vi "START_ImagenPixel.vi"() -> ()   [LabVIEW 2021]
uses:
  <vilib>/vision/NI_Vision_Development_Module.lvlib
panel:
  out "secret_in_binary":string
  out "secret_length":i32
  in  "secret_to_introduce":string
  in  "number":u8
  out "Bolean_number":bool[](array[boolean])
  out "Blue Binary":string[][](array[string])
  out "Green Number":u8[][](array[numeric])
  out "Red Number":u8[][](array[numeric])
  out "Blue Number":u8[][](array[numeric])
  out "Green Binary":string[][](array[string])
  out "Red Binary":string[][](array[string])
  out "error":errorcluster
  out "Resolution":i32[](array[numeric])
  out "Image":T1(plugin-control)
  out "Color":u32(colorbox)
  # "Image Manipulation Example"
  # "Overview: This VI creates an images from a generater random value that represents pixel RGB intensity. Afterwards, it splits the generated image again and obtains the binary values of each individual pixel and plane. \n\nRemember, for our lab, you have to ONLY MODIFY THE PIXELS IN THE RED PLANE, otherwise, the decoder won't work.\n\n\nInstructions:\n1. Set some text in secret to introduce field and Run the VI.\n2. Red Number [0][0] --> represents the amount of red color in pixel [0][0]\n2. Green Number [0][0] --> represents the amount of green color in pixel [0][0]\n2. Blue Number [0][0] --> represents the amount of blue color in pixel [0][0]\n3. Red Number [0][1] --> represents the amount of red color in pixel [0][1]\n4.All arrays have 2 dimensions as the image is a matrix of pixels\n5. Red Binary [0][0]--> Represents the value of Red Number [0][0] in binary\n6. Secret_in_binary represents the text in secret_to_introduce field in binary. Remember that each char has its own ascii equivalent\nt for example = 0b01110100\n\n\nAuthor: Jaime Burbano V\nLast Modified: 2022-06-22"
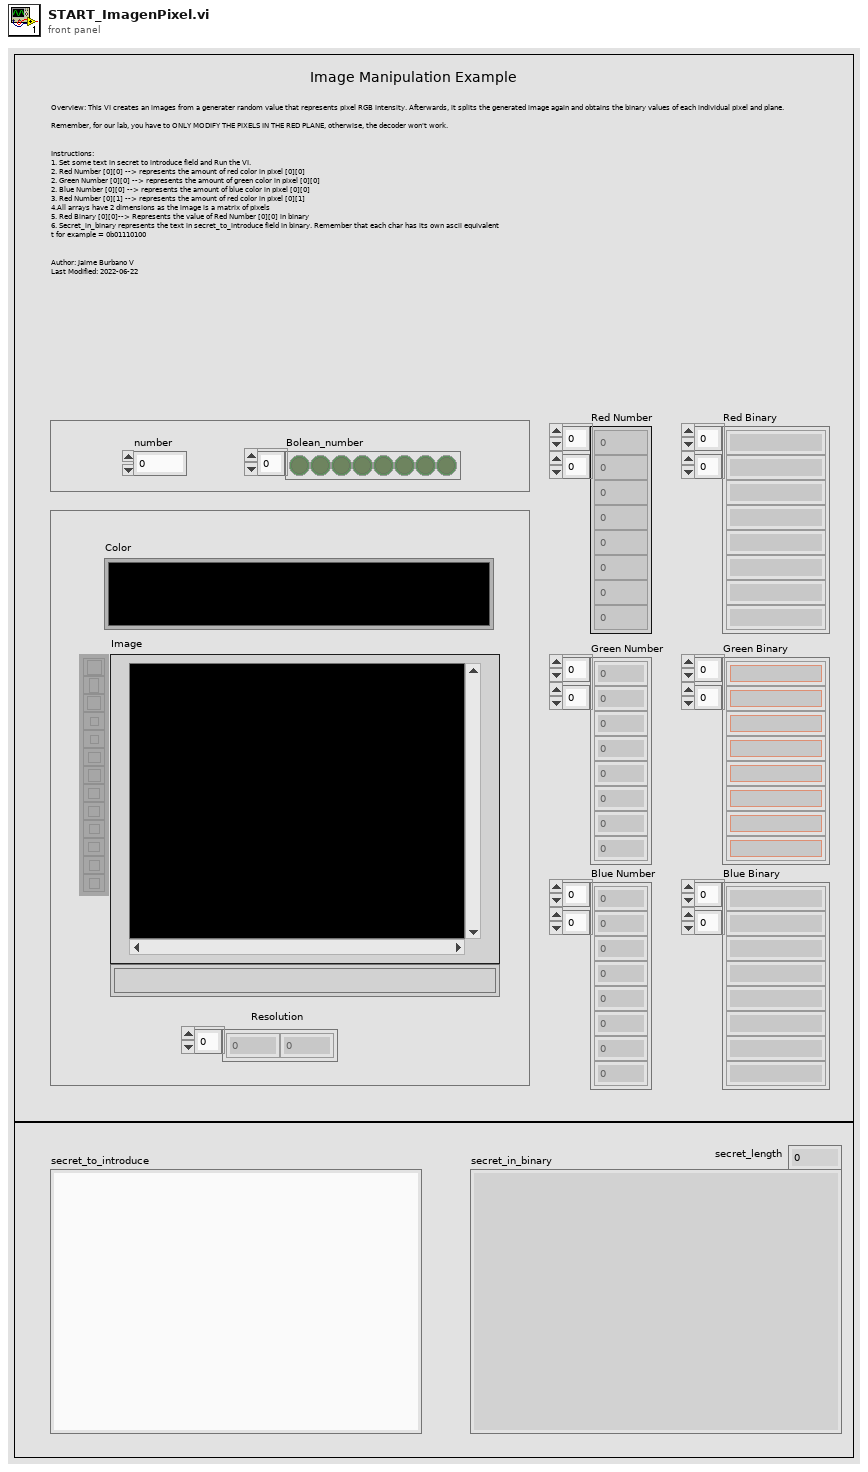
[diagram p1: front panel]
types:
  T1 = typedef "IMAQ Image.ctl" = refnum<image>
  T2 = typedef "Image Type" = u32
  T3 = cluster{"Red (or Hue) value":u8, "Green (or Sat) value":u8, "Blue (or Light or Val) value":u8}
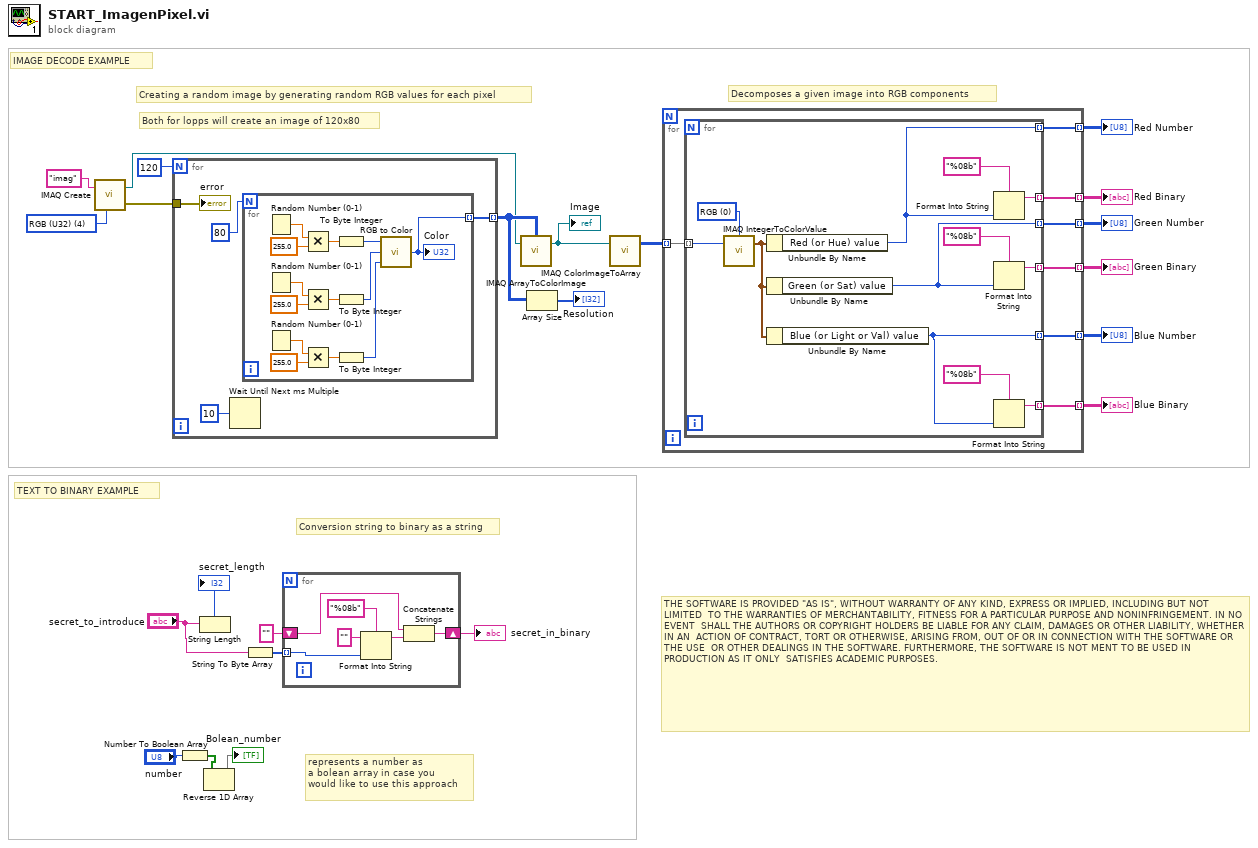
[diagram p0: block diagram]
diagram:
  w21 = T2 4 items=["Grayscale (U8)", "Grayscale (I16)", "Grayscale (SGL)", "Complex (CSG)", "RGB (U32)", "HSL (U32)", "RGB (U64)", "Grayscale (U16)"] ("Image Type")
  # "TEXT TO BINARY EXAMPLE"
  # "IMAGE DECODE EXAMPLE"
  # "Both for lopps will create an image of 120x80"
  # "THE SOFTWARE IS PROVIDED \"AS IS\", WITHOUT WARRANTY OF ANY KIND, EXPRESS OR IMPLIED, INCLUDING BUT NOT LIMITED  TO THE WARRANTIES OF MERCHANTABILITY, FITNESS FOR A PARTICULAR PURPOSE AND NONINFRINGEMENT. IN NO EVENT  SHALL THE AUTHORS OR COPYRIGHT HOLDERS BE LIABLE FOR ANY CLAIM, DAMAGES OR OTHER LIABILITY, WHETHER IN AN  ACTION OF CONTRACT, TORT OR OTHERWISE, ARISING FROM, OUT OF OR IN CONNECTION WITH THE SOFTWARE OR THE USE  OR OTHER DEALINGS IN THE SOFTWARE. FURTHERMORE, THE SOFTWARE IS NOT MENT TO BE USED IN PRODUCTION AS IT ONLY  SATISFIES ACADEMIC PURPOSES."
  # "Conversion string to binary as a string"
  # "represents a number as\na bolean array in case you \nwould like to use this approach"
  # "Decomposes a given image into RGB components"
  # "Creating a random image by generating random RGB values for each pixel"
  n1 = call "IMAQ Create"("Image Name"="imag", "Image Type"=w21) -> ("New Image"=w17:T1, "error out"=w18:errorcluster)  [unwired: 3 in]
  n2 = for {
    N: 120 -> [_]
    tunnel: [w26] -> w20 mode=indexing
    tunnel: w18 -> [w24]
    n3 = Wait Until Next ms Multiple(millisecond multiple=u32 10) -> ()  [unwired: 1 out]
    n4 = for {
      N: 80 -> [_]
      tunnel: [w28] -> w26 mode=indexing
      n5 = Random Number (0-1)() -> (number: 0 to 1=w40:dbl)
      n6 = Random Number (0-1)() -> (number: 0 to 1=w37:dbl)
      n7 = Random Number (0-1)() -> (number: 0 to 1=w36:dbl)
      n8 = Multiply(x=w40, y=255.0) -> (x*y=w34:dbl)
      n9 = Multiply(x=w37, y=255.0) -> (x*y=w33:dbl)
      n10 = Multiply(x=w36, y=255.0) -> (x*y=w32:dbl)
      n11 = To Byte Integer(number=w34) -> (8bit integer=w29:i8)
      n12 = To Byte Integer(number=w33) -> (8bit integer=w30:i8)
      n13 = To Byte Integer(number=w32) -> (8bit integer=w31:i8)
      n14 = call <vilib>:"RGB to Color.vi"("B"=w31, "G"=w30, "R"=w29) -> ("Color"=w28:u32)
      "Color" <- w28
    }
    "error" <- w24
  }
  n15 = Number To Boolean Array(number="number") -> (Boolean array=w7:bool[])
  n16 = String Length(string="secret_to_introduce") -> (length=→"secret_length":i32)
  n17 = Reverse 1D Array(array=w7) -> (reversed array=→"Bolean_number":bool[])
  n18 = String To Byte Array(string="secret_to_introduce") -> (unsigned byte array=w4:u8[])
  n19 = for {
    tunnel: w4 -> [w45] mode=indexing
    shift-right: [w43] -> w3
    shift-left: "" -> [w44]
    n20 = Format Into String(format string="%08b", initial string="", w45) -> (resulting string=w42:string)  [unwired: 1 in, 1 out]
    n21 = Concatenate Strings(w44, w42) -> (w43:string)
  }
  "secret_in_binary" <- w3
  n22 = call "IMAQ ArrayToColorImage"("Image Pixels (U32)"=w20, "Image"=w17) -> ("Image Out"=w9:T1)  [unwired: 3 in, 1 out]
  "Image" <- w9
  n23 = Array Size(array=w20) -> (size(s)=→"Resolution":i32[])
  n24 = call "IMAQ ColorImageToArray"("Image"=w9) -> ("Image Pixels (U32)"=w10:u32[][])  [unwired: 3 in, 2 out]
  n25 = for {
    tunnel: [w53] -> w13 mode=indexing
    tunnel: [w52] -> w12 mode=indexing
    tunnel: [w51] -> w14 mode=indexing
    tunnel: [w50] -> w16 mode=indexing
    tunnel: [w49] -> w15 mode=indexing
    tunnel: [w48] -> w11 mode=indexing
    tunnel: w10 -> [w47] mode=indexing
    n26 = for {
      tunnel: [w60] -> w53 mode=indexing
      tunnel: [w61] -> w52 mode=indexing
      tunnel: [w54] -> w51 mode=indexing
      tunnel: [w59] -> w50 mode=indexing
      tunnel: [w58] -> w49 mode=indexing
      tunnel: [w57] -> w48 mode=indexing
      tunnel: w47 -> [w56] mode=indexing
      w55 = u16 0 items=["RGB", "HSL", "HSV", "HSI"] ("Color Mode")
      n27 = call "IMAQ IntegerToColorValue"("U32 value"=w56, "Color Mode"=w55) -> ("Color Value"=w65:T3)  [unwired: 3 in, 3 out]
      n28 = Unbundle By Name(w65) -> ("Red (or Hue) value"=w60:u8)
      n29 = Unbundle By Name(w65) -> ("Green (or Sat) value"=w61:u8)
      n30 = Unbundle By Name(w65) -> ("Blue (or Light or Val) value"=w54:u8)
      n31 = Format Into String(format string="%08b", w60) -> (resulting string=w59:string)  [unwired: 2 in, 1 out]
      n32 = Format Into String(format string="%08b", w61) -> (resulting string=w58:string)  [unwired: 2 in, 1 out]
      n33 = Format Into String(format string="%08b", w54) -> (resulting string=w57:string)  [unwired: 2 in, 1 out]
    }
  }
  "Red Binary" <- w16
  "Green Binary" <- w15
  "Blue Number" <- w14
  "Red Number" <- w13
  "Green Number" <- w12
  "Blue Binary" <- w11
